vi "CalculoOndaContinua.vi"(0 "OndaIn":cluster{"X":dbl, "Y":dbl}[](array[cluster]), 1 "PicoMax":dbl) -> (7 "OndaOut":cluster{"X":dbl, "Y":dbl}[](graph))   [LabVIEW 2019]
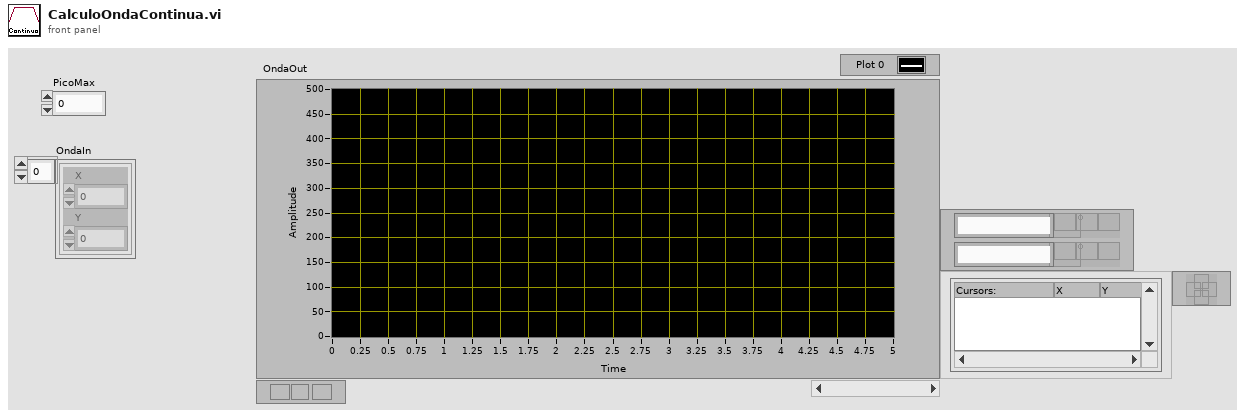
[diagram p1: front panel]
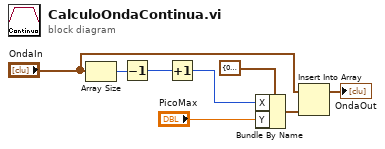
[diagram p0: block diagram]
diagram:
  n1 = Array Size(array="OndaIn") -> (size(s)=w6:i32)
  n2 = Decrement(x=w6) -> (x-1=w5:i32)
  n3 = Increment(x=w5) -> (x+1=w7:i32)
  n4 = Bundle By Name(cluster=cluster{"X":dbl, "Y":dbl} {"X"=0.0, "Y"=0.0} ("new element/subarray"), "X"=w7, "Y"="PicoMax") -> (w2:cluster{"X":dbl, "Y":dbl})
  n5 = Insert Into Array(array="OndaIn", new element=w2) -> (→"OndaOut":cluster{"X":dbl, "Y":dbl}[])  [unwired: 1 in]
